vi "cmd_scan_output_list.vi"(8 "error in (no error)":errorcluster, 11 "JSON":string) -> (0 "error out":errorcluster)   [LabVIEW 2021]
doc: "Performs a scan using a file\n \n :param filename: Specifies the file name which include output data\n :param avg: Specifies an averaged count"
uses:
  fpga/fpga_dtype_scan_config.ctl
  fpga/fpga_dtype_sgl_8ch.ctl
  core/host_global_vars.vi
panel:
  out "data":i32[](array[numeric])
  in  "args":cluster{"filename":string, "avg":i32}
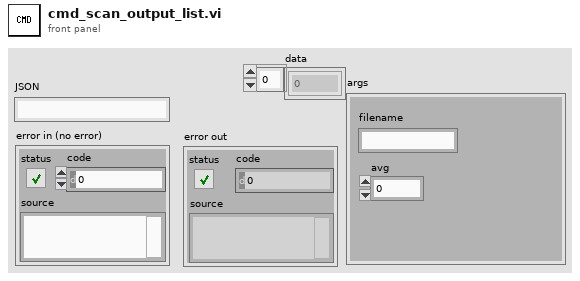
[diagram p1: front panel]
types:
  T1 = typedef "fpga_dtype_sgl_8ch.ctl" = cluster{"ch 0":sgl, "ch 1":sgl, "ch 2":sgl, "ch 3":sgl, "ch 4":sgl, "ch 5":sgl, "ch 6":sgl, "ch 7":sgl}
  T2 = typedef "fpga_dtype_scan_config.ctl" = cluster{"data points":i16, "average counts":i16, "delta per point":T1, "bidirectional scan":bool, "auto reversal":bool}
  T3 = enum16{"big-endian, network order", "native, host order", "little-endian"}
  T4 = cluster{"[0]":sgl, "[1]":sgl, "[2]":sgl, "[3]":sgl, "[4]":sgl, "[5]":sgl, "[6]":sgl, "[7]":sgl}
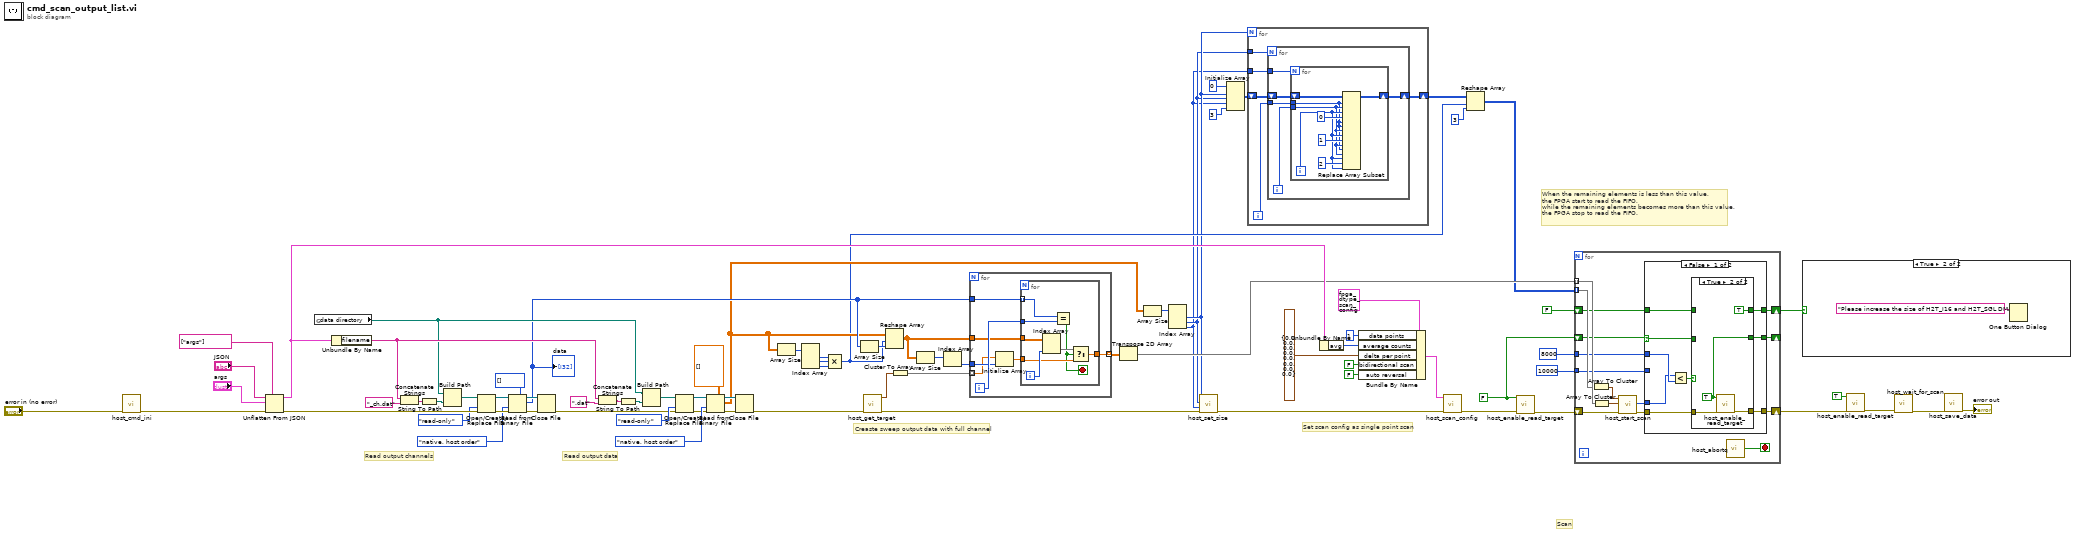
[diagram p0: block diagram]
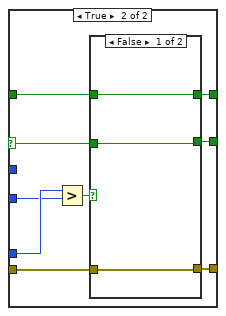
[diagram p4: hidden frame]
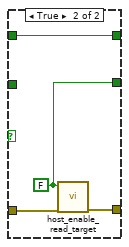
[diagram p5: hidden frame]
diagram:
  w8 = FALSE ("hold")
  # "When the remaining elements is less than this value,\nthe FPGA start to read the FIFO, \nwhile the remaining elements becomes more than this value,\nthe FPGA stop to read the FIFO."
  # "Scan"
  # "Set scan config as single point scan"
  # "Creaste sweep output data with full channel"
  # "Read output data"
  # "Read output channels"
  n1 = call "host_cmd_ini.vi"("error in (no error)"="error in (no error)") -> ("error out"=w24:errorcluster)  [unwired: 10 in]
  n2 = Unflatten From JSON(path=string[] ["args"], JSON string="JSON", type and defaults="args", error in (no error)=w24) -> (value=w39:cluster{"filename":string, "avg":i32}, error out=w69:errorcluster)  [unwired: 3 in]
  n3 = global read "host_global_vars.vi" "data directory"() -> (w52:path)
  n4 = Unbundle By Name(w39) -> ("filename"=w53:string)
  n5 = Concatenate Strings(w53, "_ch.dat") -> (w73:string)
  n6 = String To Path(string=w73) -> (path=w74:path)
  n7 = Build Path(base path=w52, name or relative path=w74) -> (appended path=w72:path)
  n8 = Open/Create/Replace File(file path (use dialog)=w72, error in=w69, access (0:read/write)=enum16{"read/write", "read-only", "write-only"}."read-only") -> (refnum out=w71:refnum<file>, error out=w76:errorcluster)  [unwired: 3 in, 1 out]
  n9 = Read from Binary File(5:i32[] [], 8:w76, 9:T3."native, host order" ("byte order (0:big-endian, network order)"), 11:w71) -> (0:w68:errorcluster, 2:w46:i32[], 3:w67:refnum<file>)  [unwired: 2 in, 1 out]
  "data" <- w46
  n10 = Close File(refnum=w67, error in=w68) -> (error out=w54:errorcluster)  [unwired: 1 out]
  n11 = Concatenate Strings(w53, ".dat") -> (w58:string)
  n12 = String To Path(string=w58) -> (path=w57:path)
  n13 = Build Path(base path=w52, name or relative path=w57) -> (appended path=w59:path)
  n14 = Open/Create/Replace File(file path (use dialog)=w59, error in=w54, access (0:read/write)=enum16{"read/write", "read-only", "write-only"}."read-only") -> (refnum out=w60:refnum<file>, error out=w55:errorcluster)  [unwired: 3 in, 1 out]
  n15 = Read from Binary File(5:sgl[][][][] [], 8:w55, 9:T3."native, host order" ("byte order (0:big-endian, network order)"), 11:w60) -> (0:w61:errorcluster, 2:w32:sgl[][][][], 3:w62:refnum<file>)  [unwired: 2 in, 1 out]
  n16 = Close File(refnum=w62, error in=w61) -> (error out=w51:errorcluster)  [unwired: 1 out]
  n17 = Array Size(array=w32) -> (size(s)=w31:i32[])
  n18 = Index Array(array=w31) -> (element #1=w30:i32, element #2=w28:i32, element #3=w29:i32)  [unwired: 3 in]
  n19 = Compound Arithmetic op=MULTIPLY(w30, w28, w29) -> (w11:i32)
  n20 = Array Size(array=w46) -> (size(s)=w47:i32)
  n21 = call "host_get_target.vi"("error in"=w51) -> ("error out"=w25:errorcluster, "target"=w50:T1)  [unwired: 9 in]
  n22 = Reshape Array(w32, w11, w47) -> (w45:sgl[][])
  n23 = Cluster To Array(cluster=w50) -> (array=w49:sgl[])
  n24 = Array Size(array=w45) -> (size(s)=w44:i32[])
  n25 = Index Array(array=w44) -> (element=w43:i32)  [unwired: 1 in]
  n26 = for {
    tunnel: w49 -> [w82] mode=indexing
    tunnel: w46 -> [w86]
    tunnel: w45 -> [w84]
    tunnel: w43 -> [w83]
    tunnel: [w80] -> w27 mode=indexing
    i -> [w85]
    n27 = Initialize Array(w82, w83) -> (w81:sgl[])
    n28 = for {
      tunnel: w86 -> [w94] mode=indexing
      tunnel: w85 -> [w93]
      tunnel: w84 -> [w92]
      tunnel: w81 -> [w89]
      tunnel: [w88] -> w80
      i -> [w91]
      stop <- w87 stop-if-true
      n29 = Index Array(array=w92, index (col)=w91) -> (element=w90:sgl[])  [unwired: 1 in]
      n30 = Equal?(x=w94, y=w93) -> (x = y?=w87:bool)
      n31 = Select(t=w90, s=w87, f=w89) -> (s? t:f=w88:sgl[])
    }
  }
  n32 = Transpose 2D Array(2D array=w27) -> (transposed array=w13:sgl[][])
  n33 = Array Size(array=w32) -> (size(s)=w42:i32[])
  n34 = Index Array(array=w42) -> (element #1=w5:i32, element #2=w4:i32, element #3=w3:i32)  [unwired: 3 in]
  n35 = call "host_set_size.vi"("error in (no error)"=w25, "fast"=w3, "slow"=w4, "page"=w5) -> ("error out"=w26:errorcluster)  [unwired: 7 in]
  n36 = Initialize Array(i16 0 ("page"), w5, w4, w3, 3 ("dimension size")) -> (w16:i16[][][][])
  n37 = for {
    N: w5 -> [_]
    shift-right: [w98] -> w12
    shift-left: w16 -> [w99]
    tunnel: w4 -> [w96]
    tunnel: w3 -> [w95]
    i -> [w97]
    n38 = for {
      N: w96 -> [_]
      shift-right: [w103] -> w98
      shift-left: w99 -> [w104]
      tunnel: w97 -> [w102]
      tunnel: w95 -> [w100]
      i -> [w101]
      n39 = for {
        N: w100 -> [_]
        shift-right: [w111] -> w103
        shift-left: w104 -> [w112]
        tunnel: w102 -> [w105]
        tunnel: w101 -> [w106]
        i -> [w107]
        n40 = Replace Array Subset(array=w112, new element #1=w105, index (dim 0) #1=w105, index (dim 1) #1=w106, index (dim 2) #1=w107, index (dim 3) #1=0 ("disabled index (col)"), new element #2=w106, index (dim 0) #2=w105, index (dim 1) #2=w106, index (dim 2) #2=w107, index (dim 3) #2=1 ("disabled index (col)"), new element #3=w107, index (dim 0) #3=w105, index (dim 1) #3=w106, index (dim 2) #3=w107, index (dim 3) #3=2 ("disabled index (col)")) -> (w111:i16[][][][])
      }
    }
  }
  n41 = Unbundle By Name(w39) -> ("avg"=w38:i32)
  n42 = Bundle By Name(cluster=T2 {"data points"=0, "average counts"=0, "delta per point"={"ch 0"=0.0, "ch 1"=0.0, "ch 2"=0.0, "ch 3"=0.0, "ch 4"=0.0, "ch 5"=0.0, "ch 6"=0.0, "ch 7"=0.0}, "bidirectional scan"=FALSE, "auto reversal"=FALSE} ("scan config"), "data points"=i16 1, "average counts"=w38, "delta per point"=T1 {"ch 0"=0.0, "ch 1"=0.0, "ch 2"=0.0, "ch 3"=0.0, "ch 4"=0.0, "ch 5"=0.0, "ch 6"=0.0, "ch 7"=0.0}, "bidirectional scan"=FALSE, "auto reversal"=FALSE) -> (w34:T2)
  n43 = call "host_scan_config.vi"("error in"=w26, "scan config"=w34) -> ("error out"=w21:errorcluster)  [unwired: 9 in]
  n44 = Reshape Array(w12, w11, 3 ("dimension size")) -> (w10:i16[][])
  n45 = call "host_enable_read_target.vi"("error in"=w21, "enable read target?"=w8) -> ("error out"=w15:errorcluster)  [unwired: 9 in]
  n46 = for {
    shift-right: [w117] -> w14
    shift-left: w15 -> [w126]
    tunnel: w13 -> [w125] mode=indexing
    tunnel: w10 -> [w124] mode=indexing
    shift-right: [w116] -> _
    shift-left: w8 -> [w121]
    tunnel: u32 10000 ("y") -> [w118]
    tunnel: u32 8000 ("y") -> [w115]
    shift-right: [w113] -> w1
    shift-left: FALSE ("hold") -> [w114]
    stop <- w127 stop-if-true
    n47 = Array To Cluster(array=w124) -> (cluster=w123:cluster{"[0]":i16, "[1]":i16, "[2]":i16})
    n48 = Array To Cluster(array=w125) -> (cluster=w122:T4)
    n49 = call "host_start_scan.vi"("error in"=w126, "initial positions"=w122, "index offset"=w123) -> ("error out"=w120:errorcluster, "Empty Elements Remaining"=w119:u32)  [unwired: 6 in, 1 out]
    n50 = case shown="False" w121 {
      selector: w121 -> [w130 w146]
      tunnel: w120 -> [w132 w148]
      tunnel: w119 -> [w135 w152]
      tunnel: w118 -> [_ w151]
      tunnel: [w133 w149] -> w117
      tunnel: [w131 w147] -> w116
      tunnel: w115 -> [w136 _]
      tunnel: w114 -> [w129 w144]
      tunnel: [w128 w145] -> w113
      frame False {
        n51 = Less?(x=w135, y=w136) -> (x < y?=w134:bool)
        n52 = case shown="True" w134 {
          tunnel: [w138 w143] -> w133
          tunnel: w132 -> [w138 w142]
          tunnel: [w139 w141] -> w131
          tunnel: w130 -> [w139 _]
          tunnel: w129 -> [w137 _]
          tunnel: [w137 TRUE ("hold")] -> w128
          frame False {
          }
          frame True {
            w141 = TRUE ("enable read target?")
            n53 = call "host_enable_read_target.vi"("error in"=w142, "enable read target?"=w141) -> ("error out"=w143:errorcluster)  [unwired: 9 in]
          }
        }
      }
      frame True {
        n54 = Greater?(x=w152, y=w151) -> (0:w150:bool)
        n55 = case shown="False" w150 {
          tunnel: [w154 w159] -> w149
          tunnel: w148 -> [w154 w158]
          tunnel: [w155 w157] -> w147
          tunnel: w146 -> [w155 _]
          tunnel: [w153 w156] -> w145
          tunnel: w144 -> [w153 w156]
          frame False {
          }
          frame True {
            w157 = FALSE ("enable read target?")
            n56 = call "host_enable_read_target.vi"("error in"=w158, "enable read target?"=w157) -> ("error out"=w159:errorcluster)  [unwired: 9 in]
          }
        }
      }
    }
    n57 = call "host_abortq.vi"() -> ("abort"=w127:bool)  [unwired: 1 in]
  }
  n58 = case shown="True" w1 {
    frame False {
    }
    frame True {
      n59 = One Button Dialog(message="Please increase the size of H2T_I16 and H2T_SGL DMA") -> ()  [unwired: 1 in, 1 out]
    }
  }
  n60 = call "host_enable_read_target.vi"("error in"=w14, "enable read target?"=TRUE ("hold")) -> ("error out"=w20:errorcluster)  [unwired: 9 in]
  n61 = call "host_wait_for_scan.vi"("error in (no error)"=w20) -> ("error out"=w22:errorcluster)  [unwired: 10 in]
  n62 = call "host_save_data.vi"("error in"=w22) -> ("error out"=→"error out":errorcluster)  [unwired: 10 in]
